vi "Calculate Permutations from Combinations.vi"(10 "Solutions":i32[][](array[numeric]), 11 "Quantity":i32[](array[numeric])) -> (2 "How many permutations":dbl, 3 "binomial coefficient (n,k)":dbl=1.0)   [LabVIEW 2014]
uses:
  <vilib>/gmath/NI_Gmath.lvlib
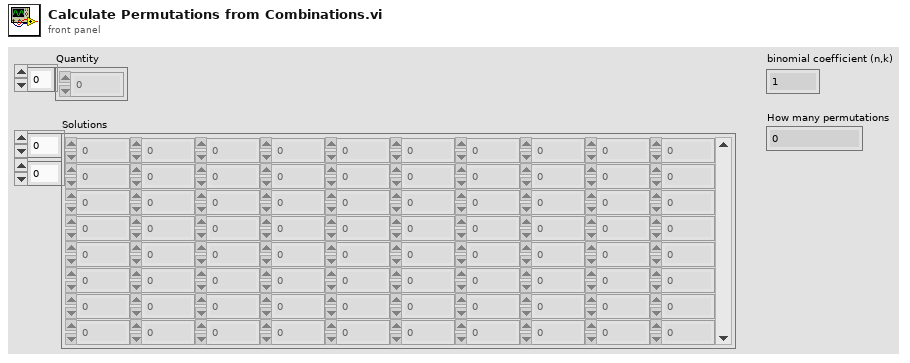
[diagram p1: front panel]
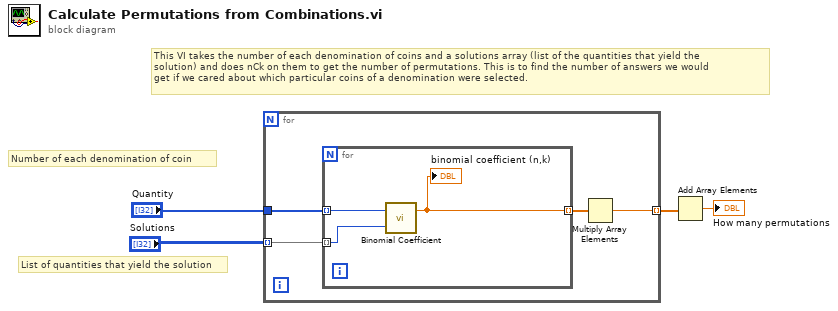
[diagram p0: block diagram]
diagram:
  # "List of quantities that yield the solution"
  # "Number of each denomination of coin"
  # "This VI takes the number of each denomination of coins and a solutions array (list of the quantities that yield the\nsolution) and does nCk on them to get the number of permutations. This is to find the number of answers we would \nget if we cared about which particular coins of a denomination were selected."
  n1 = for {
    tunnel: "Solutions" -> [w8] mode=indexing
    tunnel: "Quantity" -> [w7]
    tunnel: [w5] -> w1 mode=indexing
    n2 = for {
      tunnel: w8 -> [w11] mode=indexing
      tunnel: w7 -> [w10] mode=indexing
      tunnel: [w9] -> w6 mode=indexing
      n3 = call <vilib>:"Binomial Coefficient.vi"("k"=w11, "n"=w10) -> ("binomial coefficient (n,k)"=w9:dbl)  [unwired: 1 out]
      "binomial coefficient (n,k)" <- w9
    }
    n4 = Multiply Array Elements(1:w6) -> (0:w5:dbl)
  }
  n5 = Add Array Elements(numeric array=w1) -> (sum=→"How many permutations":dbl)
